vi "Main.vi"() -> ()   [LabVIEW 2016]
uses:
  <vilib>/NXT/Subs/ColorSensorColors.ctl
  <vilib>/NXT/LegoClasses/BrickReference/BrickReference.lvclass
  <vilib>/NXT/Subs/LVHSConnector.ctl
  booleanos.ctl
  caracteristicas.ctl
  <vilib>/NXT/Block Support/NXT_InputPort.ctl
  parametros.ctl
panel:
  out "Direct bool":bool
  in  "Parâmetros Iniciais":T1={"Gyro Port"=0, "Sensor - Left"=3, "Sensor - Right"=2, "     Color \nSensor Port"=1, "Kp Front"=0.6, "Motor speed"=-15, "Distance to street"=20.0, "Motor speed turns"=16, "Kp Curvas"=0.3} {"Kp Front" format="%.3f"; "Color \nSensor Port" items=["Port 1", "Port 2", "Port 3", "Port 4"]; "Sensor - Right" items=["Port 1", "Port 2", "Port 3", "Port 4"]; "Sensor - Left" items=["Port 1", "Port 2", "Port 3", "Port 4"]; "Gyro Port" items=["Port 1", "Port 2", "Port 3", "Port 4"]}
  in  "Características Iniciais":T3={"Colors and Directions"=[enum."Zero", enum."Zero", enum."Zero", enum."Zero", enum."Zero", enum."Zero"], "Direction"=enum."Zero", "CS"=enum."Street", "Old Color"=enum."White"}
  in  "Booleanos e Contadores \nIniciais":T5={"Correct"=FALSE, "Enable State change"=TRUE, "First End"=FALSE, "Intersections crossed"=0.0, "Intersections crossed total"=0.0, "Bonecos"=0.0, "Inter correct"=FALSE} caption="Booleanos e Contadores"
  out "NXT/EV3 2":T6
  in  "NXT/EV3":T6
  # "black"
  # "blue"
  # "green"
  # "yellow"
  # "red"
  # "Permite que ocorra troca \nde estados se True e interrompe-as \nse False."
  # "Booleano que retorna F quando chega em Delivery.\nGarantindo que não contará\nmais intersections"
  # "Salva o total de interseções \ncruzadas"
  # "Contador de quantas \ninterseções foram cruzadas.\nSoma ao acertar"
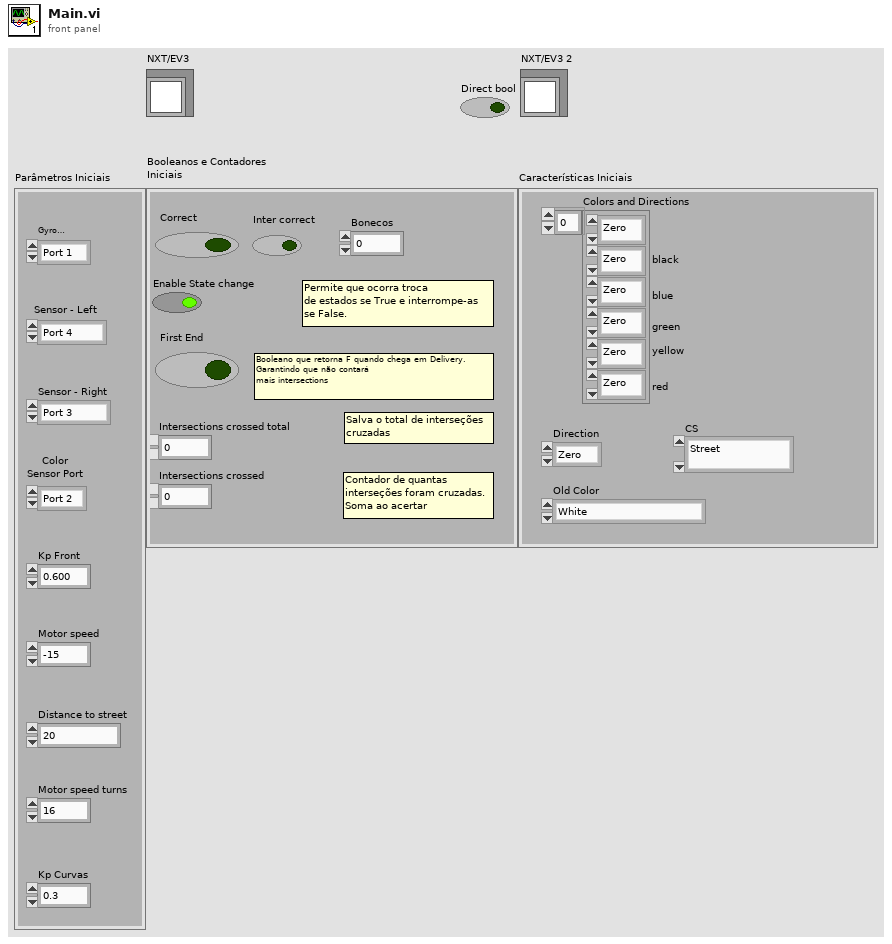
[diagram p1: front panel]
types:
  T1 = typedef "parametros.ctl" = cluster{"Gyro Port":T2, "Sensor - Left":T2, "Sensor - Right":T2, "     Color \nSensor Port":T2, "Kp Front":dbl, "Motor speed":i32, "Distance to street":dbl, "Motor speed turns":i32, "Kp Curvas":dbl}
  T2 = typedef "NXT_InputPort.ctl" = u32
  T3 = typedef "caracteristicas.ctl" = cluster{"Colors and Directions":enum16{"Zero", "Right", "Front", "Left"}[], "Direction":enum16{"Zero", "Right", "Front", "Left"}, "CS":enum16{"Street", "Intersection", "End", "Stop", "Square", "Delivery", "Empty"}, "Old Color":T4}
  T4 = typedef "ColorSensorColors.ctl" = enum16{"No Color", "Black", "Blue", "Green", "Yellow", "Red", "White", "Brown"}
  T5 = typedef "booleanos.ctl" = cluster{"Correct":bool, "Enable State change":bool, "First End":bool, "Intersections crossed":dbl, "Intersections crossed total":dbl, "Bonecos":dbl, "Inter correct":bool}
  T6 = typedef "LVHSConnector.ctl" = refnum<class "BrickReference.lvclass">
  T7 = enum16{"Street", "Intersection", "End", "Stop", "Square", "Delivery", "Empty"}
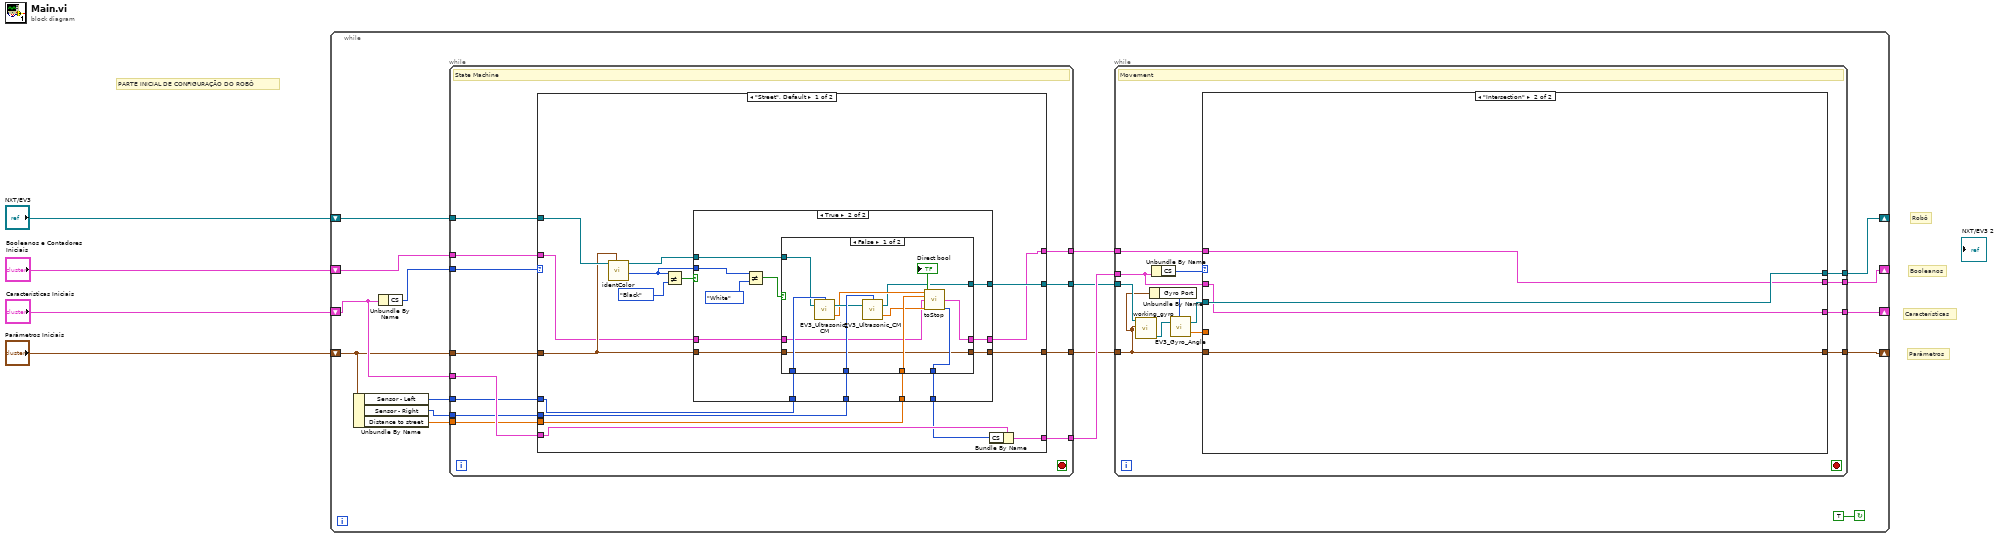
[diagram p0: block diagram]
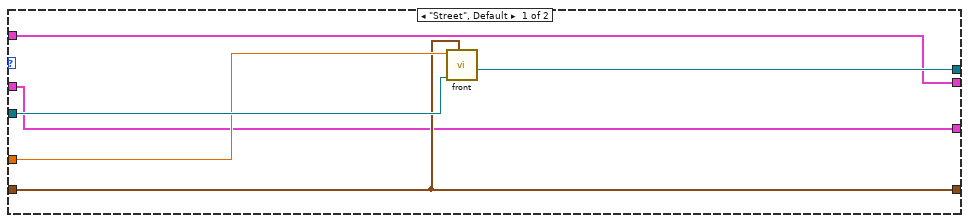
[diagram p2: hidden frame]
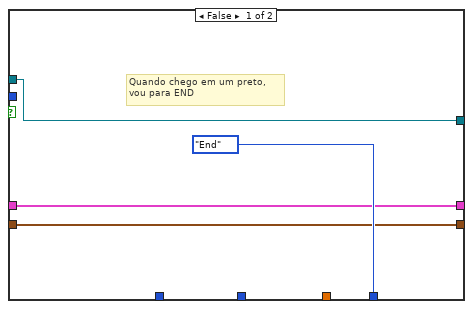
[diagram p3: hidden frame]
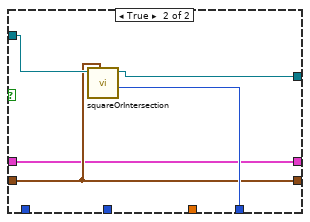
[diagram p4: hidden frame]
diagram:
  # "Booleanos"
  # "Robô"
  # "Parâmetros"
  # "Características"
  # "PARTE INICIAL DE CONFIGURAÇÃO DO ROBÔ"
  n1 = while {
    shift-right: [w9] -> _
    shift-left: "NXT/EV3" -> [w17]
    shift-right: [w6] -> _
    shift-left: "Booleanos e Contadores \nIniciais" -> [w12]
    shift-right: [w7] -> _
    shift-left: "Características Iniciais" -> [w19]
    shift-right: [w8] -> _
    shift-left: "Parâmetros Iniciais" -> [w16]
    stop <- TRUE continue-if-true
    n2 = Unbundle By Name(w16) -> ("Sensor - Left"=w14:T2, "Sensor - Right"=w13:T2, "Distance to street"=w15:dbl)
    n3 = Unbundle By Name(w19) -> ("CS"=w20:T7)
    n4 = while {
      tunnel: w20 -> [w56]
      tunnel: w19 -> [w55]
      tunnel: [w54] -> w18
      tunnel: w17 -> [w53]
      tunnel: w16 -> [w52]
      tunnel: w15 -> [w51]
      tunnel: w14 -> [w50]
      tunnel: w13 -> [w49]
      tunnel: w12 -> [w48]
      tunnel: [w47] -> w11
      tunnel: [w46] -> w10
      tunnel: [w45] -> w5
      stop <- _ stop-if-true
      # "State Machine"
      n5 = case shown="\"Street\", Default" w56 {
        tunnel: w55 -> [w72 w109]
        tunnel: [w71 w109] -> w54
        tunnel: w53 -> [w70 w111]
        tunnel: w52 -> [w65 w110]
        tunnel: w51 -> [w63 _]
        tunnel: w50 -> [w62 _]
        tunnel: w49 -> [w61 _]
        tunnel: w48 -> [w60 w108]
        tunnel: [w59 w111] -> w47
        tunnel: [w58 w110] -> w46
        tunnel: [w57 w108] -> w45
        frame "Street", Default {
          n6 = call "identColor.vi"("Parâmetros Ini"=w65, "NXT/EV3"=w70) -> ("Collor"=w66:T4, "NXT/EV3 2"=w64:T6)  [unwired: 8 in]
          n7 = Not Equal?(x=w66, y=ColorSensorColors."Black") -> (x != y?=w68:bool)
          n8 = case shown="True" w68 {
            tunnel: [T7."End" ("CS") w84] -> w67
            tunnel: w66 -> [_ w89]
            tunnel: w65 -> [w74 w86]
            tunnel: w64 -> [w75 w85]
            tunnel: w63 -> [_ w83]
            tunnel: w62 -> [_ w82]
            tunnel: w61 -> [_ w81]
            tunnel: w60 -> [w73 w80]
            tunnel: [w75 w79] -> w59
            tunnel: [w74 w78] -> w58
            tunnel: [w73 w77] -> w57
            frame False {
              # "Quando chego em um preto,\nvou para END"
            }
            frame True {
              n9 = Not Equal?(x=w89, y=ColorSensorColors."White") -> (x != y?=w87:bool)
              n10 = case shown="False" w87 {
                tunnel: w86 -> [w92 w104]
                tunnel: w85 -> [w99 w107]
                tunnel: [w95 w106] -> w84
                tunnel: w83 -> [w102 _]
                tunnel: w82 -> [w101 _]
                tunnel: w81 -> [w100 _]
                tunnel: w80 -> [w91 w103]
                tunnel: [w93 w105] -> w79
                tunnel: [w92 w104] -> w78
                tunnel: [w90 w103] -> w77
                frame False {
                  n11 = call <vilib>:"EV3_Ultrasonic_CM.vi"("NXT/EV3"=w99, "Port (Port 1)"=w101) -> ("Centimeters"=w97:sgl, "NXT/EV3"=w98:T6)  [unwired: 1 in]
                  n12 = call <vilib>:"EV3_Ultrasonic_CM.vi"("NXT/EV3"=w98, "Port (Port 1)"=w100) -> ("Centimeters"=w96:sgl, "NXT/EV3"=w93:T6)  [unwired: 1 in]
                  n13 = call "toStop.vi"("Left"=w97, "Distance to street"=w102, "Booleanos e Contadores Iniciais IN"=w91, "Right"=w96) -> ("Boolean"=→"Direct bool":bool, "Booleanos e Contadores Iniciais OUT"=w90:T5, "CS OUT"=w95:T7)  [unwired: 8 in, 1 out]
                }
                frame True {
                  n14 = call "squareOrIntersection.vi"("Parâmetros Ini"=w104, "NXT/EV3"=w107) -> ("CS"=w106:enum16{"Street", "Intersection", "End", "Stop"}, "NXT/EV3 2"=w105:T6)  [unwired: 7 in]
                }
              }
            }
          }
          n15 = Bundle By Name(cluster=w72, "CS"=w67) -> (w71:T3)
        }
        frame "Intersection" {
        }
      }
    }
    n16 = while {
      tunnel: w18 -> [w25]
      tunnel: w11 -> [w33]
      tunnel: w10 -> [w27]
      tunnel: [w29] -> w9
      tunnel: [w28] -> w8
      tunnel: [w24] -> w7
      tunnel: [w23] -> w6
      tunnel: w5 -> [w22]
      stop <- _ stop-if-true
      # "Movement"
      n17 = call "working_gyro.vi"("Parâmetros Iniciais"=w27, "NXT/EV3"=w33) -> ("NXT/EV3 2"=w32:T6)  [unwired: 9 in]
      n18 = Unbundle By Name(w27) -> ("Gyro Port"=w30:T2)
      n19 = Unbundle By Name(w25) -> ("CS"=w34:T7)
      n20 = call <vilib>:"EV3_Gyro_Angle.vi"("NXT/EV3"=w32, "Port (Port 1)"=w30) -> ("Degrees"=w26:sgl, "NXT/EV3"=w31:T6)  [unwired: 1 in]
      n21 = case shown="\"Intersection\"" w34 {
        tunnel: w31 -> [w40 w44]
        tunnel: [w39 w44] -> w29
        tunnel: [w37 w42] -> w28
        tunnel: w27 -> [w37 w42]
        tunnel: w26 -> [w38 _]
        tunnel: w25 -> [w36 w43]
        tunnel: [w36 w43] -> w24
        tunnel: [w35 w41] -> w23
        tunnel: w22 -> [w35 w41]
        frame "Street", Default {
          n22 = call "front.vi"("Parâmetros Ini 2"=w37, "NXT/EV3"=w40, "First Angle"=w38) -> ("NXT/EV3 2"=w39:T6)  [unwired: 8 in]
        }
        frame "Intersection" {
        }
      }
    }
  }
